vi "Is DQMH module API tester.vi"(11 "File Name":string) -> (3 "Is API Tester?":bool)   [LabVIEW 2021, in "TAF Proj Document Type.lvlib"]
uses:
  <vilib>/Wovalab/AntiDoc/Document Type/Add-ons/LabVIEW TAF Project/TAF Proj Document Type.lvlib
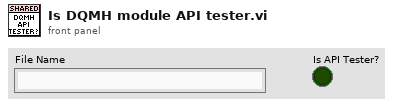
[diagram p1: front panel]
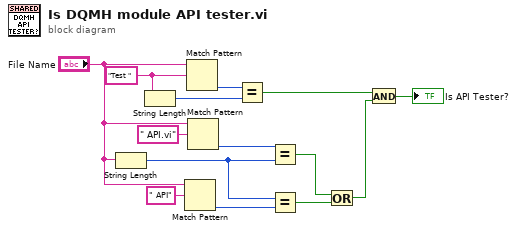
[diagram p0: block diagram]
diagram:
  w9 = "Test " ("regular expression")
  n1 = String Length(string="File Name") -> (length=w6:i32)
  n2 = String Length(string=w9) -> (length=w8:i32)
  n3 = Match Pattern(string="File Name", regular expression=" API") -> (offset past match=w7:i32)  [unwired: 4 out]
  n4 = Match Pattern(string="File Name", regular expression=w9) -> (offset past match=w10:i32)  [unwired: 4 out]
  n5 = Match Pattern(string="File Name", regular expression=" API.vi") -> (offset past match=w11:i32)  [unwired: 4 out]
  n6 = Equal?(x=w10, y=w8) -> (x = y?=w3:bool)
  n7 = Equal?(x=w11, y=w6) -> (x = y?=w5:bool)
  n8 = Equal?(x=w6, y=w7) -> (x = y?=w4:bool)
  n9 = Or(x=w5, y=w4) -> (x .or. y?=w2:bool)
  n10 = And(x=w3, y=w2) -> (x .and. y?=→"Is API Tester?":bool)
